vi "DHE_TP_parse_request.vi"(8 "error in (no error)":errorcluster, 9 "desired points":string, 10 "TPs":T1[](array[typedef]) {"Limits"."nominal" format="%.2f"; "Limits"."Lower" format="%.2f"; "Limits"."upper" format="%.2f"}) -> (0 "error out":errorcluster, 1 "indexes":i32[](array[numeric]), 2 "tps":T1[](array[typedef]) {"Limits"."nominal" format="%.2f"; "Limits"."Lower" format="%.2f"; "Limits"."upper" format="%.2f"}, 3 "number of points":i32, 4 "mult. points?":bool, 5 "found":bool)   [LabVIEW 2016]
uses:
  DHE_TP.ctl
  DHE_TPLimits.ctl
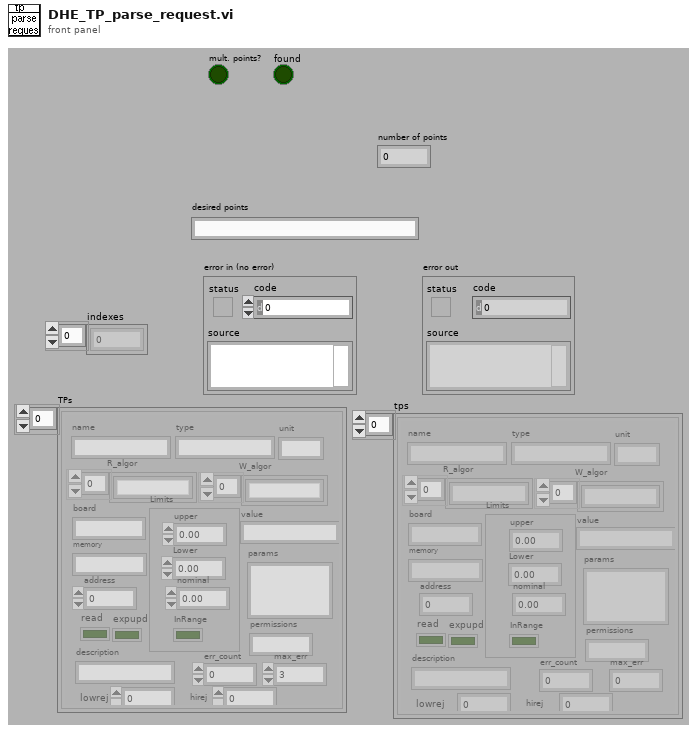
[diagram p1: front panel]
types:
  T1 = typedef "DHE_TP.ctl" = cluster{"name":string, "type":string, "R_algor":string[], "board":string, "memory":string, "address":i32, "value":string, "Limits":T2, "unit":string, "params":string, "permissions":string, "W_algor":string[], "description":string, "err_count":i32, "max_err":i32, "read":bool, "lowrej":dbl, "hirej":dbl, "expupd":bool}
  T2 = typedef "DHE_TPLimits.ctl" = cluster{"upper":dbl, "Lower":dbl, "InRange":bool, "nominal":dbl}
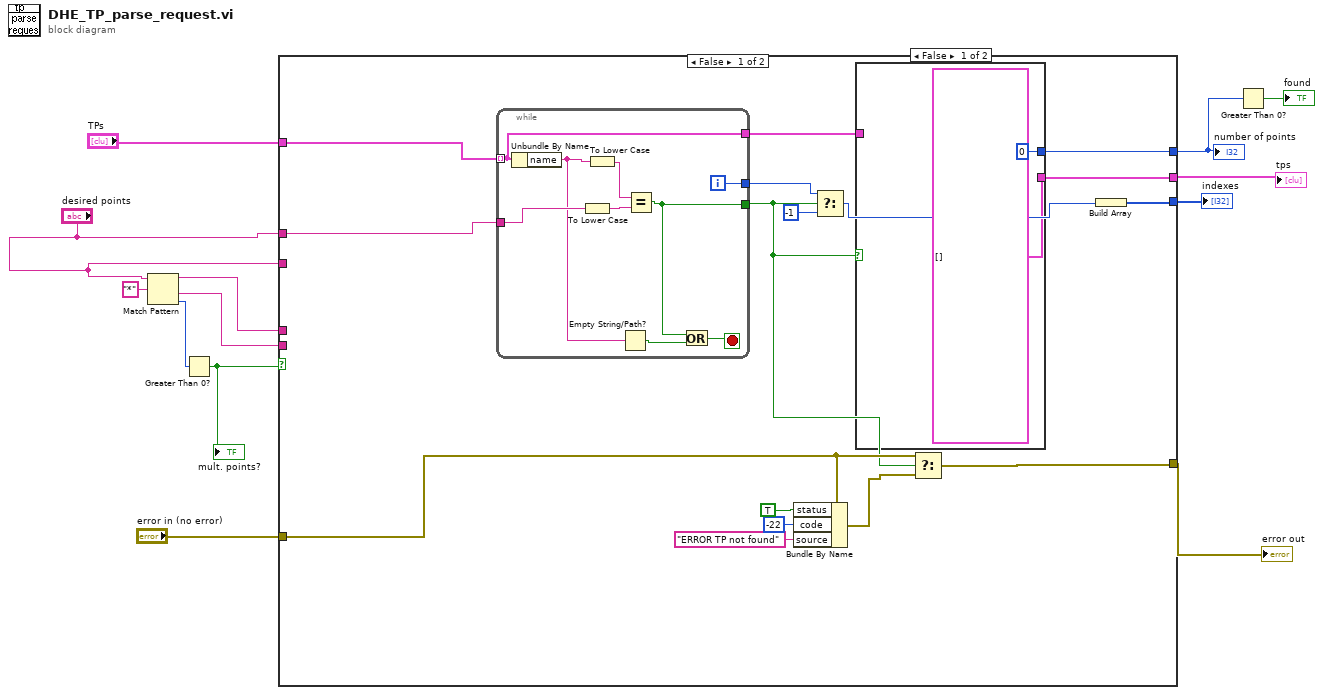
[diagram p0: block diagram]
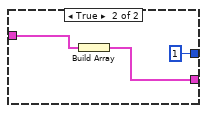
[diagram p2: hidden frame]
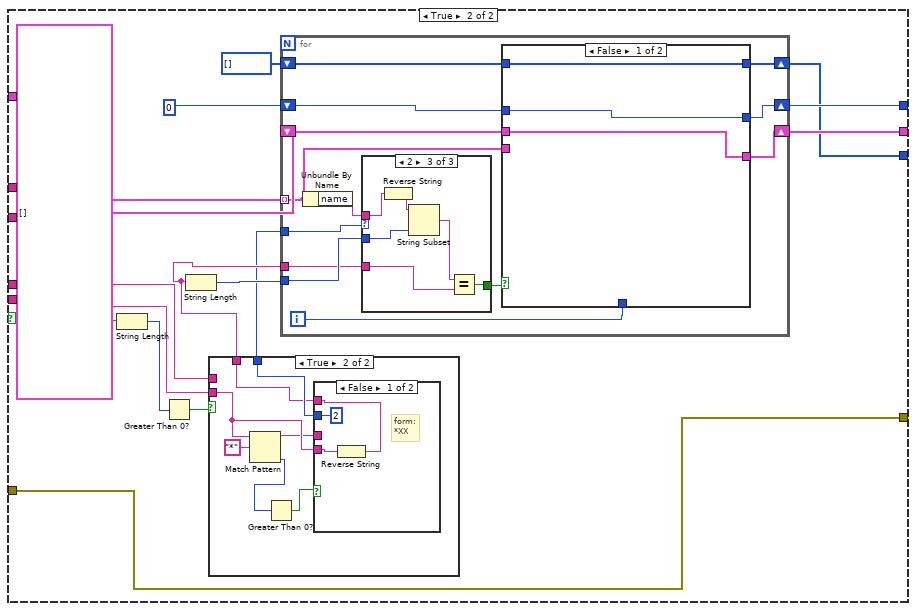
[diagram p3: hidden frame]
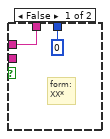
[diagram p4: hidden frame]
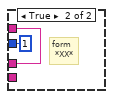
[diagram p5: hidden frame]
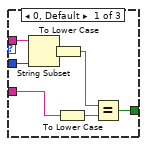
[diagram p6: hidden frame]
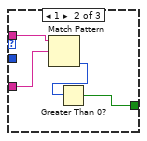
[diagram p7: hidden frame]
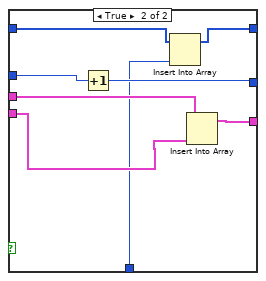
[diagram p8: hidden frame]
diagram:
  n1 = Match Pattern(string="desired points", regular expression="*") -> (before substring=w10:string, after substring=w9:string, offset past match=w12:i32)  [unwired: 2 out]
  n2 = Greater Than 0?(x=w12) -> (x > 0?=w11:bool)
  "mult. points?" <- w11
  n3 = case shown="False" w11 {
    tunnel: w10 -> [_ w54]
    tunnel: [w19 w47] -> w8
    tunnel: w9 -> [_ w55]
    tunnel: "desired points" -> [_ _]
    tunnel: "error in (no error)" -> [w29 w51]
    tunnel: [w27 w51] -> w5
    tunnel: "desired points" -> [w22 _]
    tunnel: "TPs" -> [w23 w50]
    tunnel: [w16 w48] -> w2
    tunnel: [w15 w44] -> w1
    frame False {
      n4 = while {
        tunnel: w23 -> [w35] mode=indexing
        tunnel: w22 -> [w43]
        tunnel: [w37] -> w18
        tunnel: [w36] -> w21
        tunnel: [w35] -> w17
        i -> [w36]
        stop <- w38 stop-if-true
        n5 = Unbundle By Name(w35) -> ("name"=w40:string)
        n6 = To Lower Case(string=w43) -> (all lower case string=w41:string)
        n7 = To Lower Case(string=w40) -> (all lower case string=w42:string)
        n8 = Empty String/Path?(string/path=w40) -> (empty?=w39:bool)
        n9 = Equal?(x=w42, y=w41) -> (x = y?=w37:bool)
        n10 = Or(x=w37, y=w39) -> (x .or. y?=w38:bool)
      }
      n11 = Bundle By Name(cluster=w29, "status"=TRUE, "code"=-22, "source"="ERROR TP not found") -> (w28:errorcluster)
      n12 = Select(t=w21, s=w18, f=-1) -> (s? t:f=w14:i32)
      n13 = case shown="False" w18 {
        tunnel: [0 ("t") 1 ("t")] -> w19
        tunnel: w17 -> [_ w34]
        tunnel: [T1[] [] w33] -> w16
        frame False {
        }
        frame True {
          n14 = Build Array(w34) -> (w33:T1[])
        }
      }
      n15 = Select(t=w29, s=w18, f=w28) -> (s? t:f=w27:errorcluster)
      n16 = Build Array(w14) -> (w15:i32[])
    }
    frame True {
      n17 = String Length(string=w55) -> (length=w57:i32)
      n18 = Greater Than 0?(x=w57) -> (x > 0?=w56:bool)
      n19 = case shown="True" w56 {
        tunnel: w55 -> [_ w63]
        tunnel: w54 -> [w60 _]
        tunnel: [w60 w61] -> w53
        tunnel: [0 w64] -> w52
        frame False {
          # "form:\nXX*"
        }
        frame True {
          n20 = Match Pattern(string=w63, regular expression="*") -> (before substring=w62:string, offset past match=w66:i32)  [unwired: 3 out]
          n21 = Greater Than 0?(x=w66) -> (x > 0?=w65:bool)
          n22 = case shown="False" w65 {
            tunnel: [2 1] -> w64
            tunnel: w63 -> [w69 _]
            tunnel: w62 -> [_ w71]
            tunnel: [w68 w71] -> w61
            frame False {
              # "form:\n*XX"
              n23 = Reverse String(1:w69) -> (0:w68:string)
            }
            frame True {
              # "form\n *XX*"
            }
          }
        }
      }
      n24 = String Length(string=w53) -> (length=w58:i32)
      n25 = for {
        tunnel: w53 -> [w84]
        tunnel: w58 -> [w85]
        shift-right: [w81] -> w47
        shift-left: 0 -> [w82]
        shift-right: [w80] -> w48
        shift-left: T1[] [] -> [w79]
        tunnel: w52 -> [w78]
        tunnel: w50 -> [w76] mode=indexing
        shift-right: [w74] -> w44
        shift-left: i32[] [] -> [w73]
        i -> [w75]
        n26 = Unbundle By Name(w76) -> ("name"=w77:string)
        n27 = case shown="2" w78 {
          tunnel: w85 -> [w92 _ w100]
          tunnel: w84 -> [w91 w95 w98]
          tunnel: [w90 w93 w97] -> w83
          tunnel: w77 -> [w88 w96 w102]
          frame 0, Default {
            n28 = String Subset(string=w88, length (rest)=w92) -> (substring=w89:string)  [unwired: 1 out]
            n29 = To Lower Case(string=w89) -> (all lower case string=w87:string)
            n30 = To Lower Case(string=w91) -> (all lower case string=w86:string)
            n31 = Equal?(x=w87, y=w86) -> (x = y?=w90:bool)
          }
          frame 1 {
            n32 = Match Pattern(string=w96, regular expression=w95) -> (offset past match=w94:i32)  [unwired: 4 out]
            n33 = Greater Than 0?(x=w94) -> (x > 0?=w93:bool)
          }
          frame 2 {
            n34 = Reverse String(1:w102) -> (0:w101:string)
            n35 = String Subset(string=w101, length (rest)=w100) -> (substring=w99:string)  [unwired: 1 out]
            n36 = Equal?(x=w99, y=w98) -> (x = y?=w97:bool)
          }
        }
        n37 = case shown="False" w83 {
          tunnel: w76 -> [_ w109]
          tunnel: w82 -> [w105 w113]
          tunnel: [w105 w112] -> w81
          tunnel: [w104 w111] -> w80
          tunnel: w79 -> [w104 w110]
          tunnel: w75 -> [_ w108]
          tunnel: [w103 w107] -> w74
          tunnel: w73 -> [w103 w106]
          frame False {
          }
          frame True {
            n38 = Increment(x=w113) -> (x+1=w112:i32)
            n39 = Insert Into Array(array=w106, new element=w108) -> (w107:i32[])  [unwired: 1 in]
            n40 = Insert Into Array(array=w110, new element=w109) -> (w111:T1[])  [unwired: 1 in]
          }
        }
      }
    }
  }
  "number of points" <- w8
  "error out" <- w5
  "indexes" <- w1
  "tps" <- w2
  n41 = Greater Than 0?(x=w8) -> (x > 0?=→"found":bool)
